vi "Set Comms Loop Next State.vi"(7 "Command":T1, 8 "error in (no error)":errorcluster, 11 "Data":variant) -> (0 "error out":errorcluster)   [LabVIEW 2019]
uses:
  Controls/Comms Loop States.ctl
  Controls/Comms Loop State Controller Message.ctl
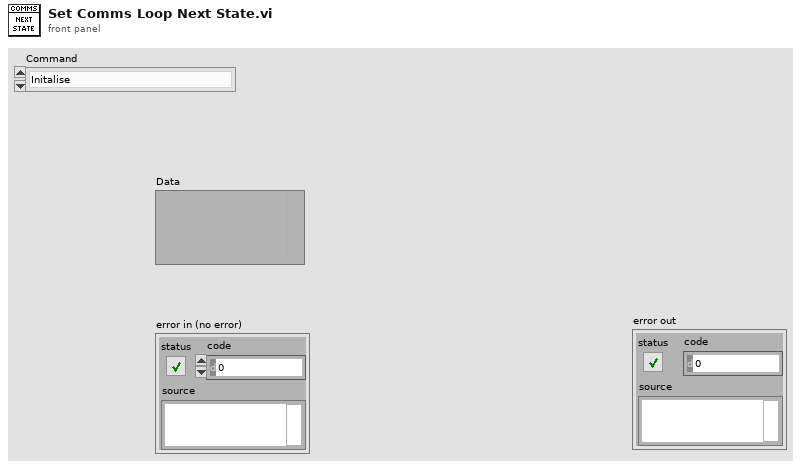
[diagram p1: front panel]
types:
  T1 = typedef "Comms Loop States.ctl" = enum16{"Initalise", "User Event", "HEART_BEAT", "SEND_LOG_FILE_NAME", "Clear Log File Names", "SEND_LOG_FILE_CHUNK", "SEND_LOG_FILE_SIZE", "SEND_SD_CARD_INFO", "SEND_BATTERY_INFO", "SEND_LOGGING_PERIOD", "SEND_RTC_TIME", "SEND_CURRENT_MEASUREMENTS", "ERROR_MSG", "Clear Error Messages", "Send Message", "Idle", "Sensor Connected", "Sensor Disconnected", "Set Page Displayed", "Set Connected Sensor Type", "UI: Update Sensor Type", "UI: Update Log List", "Reset Log File Transfer", "SEND_WIFI_DETAILS", "Complete Transfer"}
  T2 = typedef "Comms Loop State Controller Message.ctl" = cluster{"Command":T1, "Data":variant}
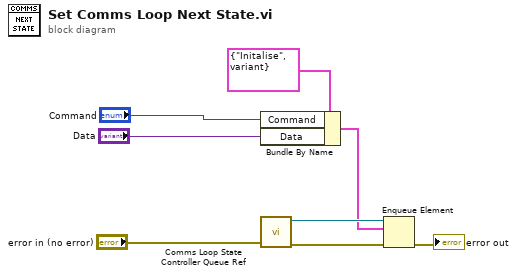
[diagram p0: block diagram]
diagram:
  n1 = Bundle By Name(cluster=T2 {"Command"=enum."Initalise", "Data"=variant} ("element"), "Command"="Command", "Data"="Data") -> (w2:T2)
  n2 = call "Comms Loop State Controller Queue Ref.vi"("error in (no error)"="error in (no error)") -> ("error out"=w6:errorcluster, "queue out"=w5:refnum<queue>)  [unwired: 9 in]
  n3 = Enqueue Element(queue=w5, element=w2, error in (no error)=w6) -> (error out=→"error out":errorcluster)  [unwired: 1 in, 2 out]
